vi "testInternalMemoryDispose.vi"(8 "error in (no error)":errorcluster, 11 "TestCase in":refnum<class "Memory Manager Unit Tests.lvclass">) -> (0 "error out":errorcluster, 3 "TestCase out":refnum<class "Memory Manager Unit Tests.lvclass">)   [LabVIEW 2016, in "Memory Manager Unit Tests.lvclass"]
uses:
  Memory Manager Unit Tests.lvclass
  Library/Classes/Pointer.Internal/Memory.Pointer.Internal.lvclass
  C:/Git/Personal/LabVIEW-Memory-Manager/Source/Library/Classes/Pointer/Memory.Pointer.lvclass
  Library/Classes/Pointer/Memory.Pointer.lvclass/Memory.Pointer.ctl
  Library/Classes/Pointer/Accessors/Get Address.vi
  <vilib>/addons/_JKI Toolkits/VI Tester/TestCase.llb/TestCase.lvclass
  C:/Program Files (x86)/National Instruments/LabVIEW 2016/vi.lib/addons/_JKI Toolkits/VI Tester/TestCase.llb/TestCase.lvclass
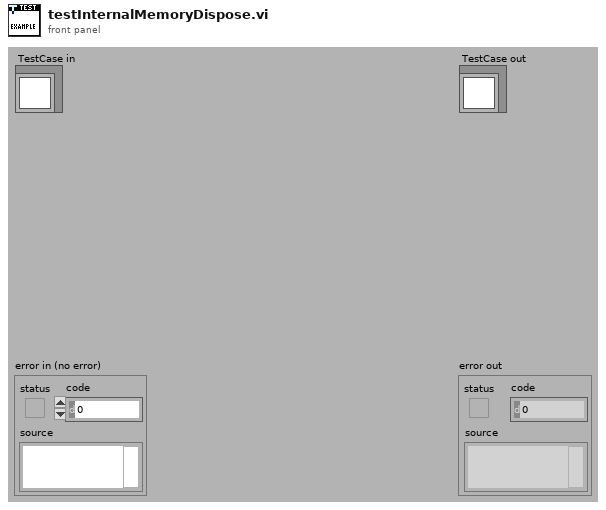
[diagram p1: front panel]
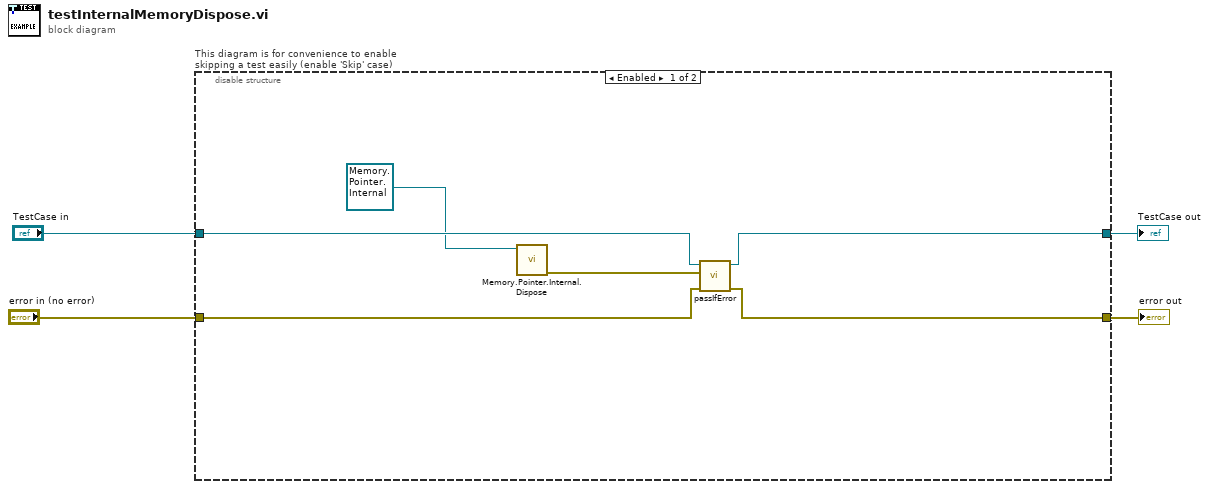
[diagram p0: block diagram]
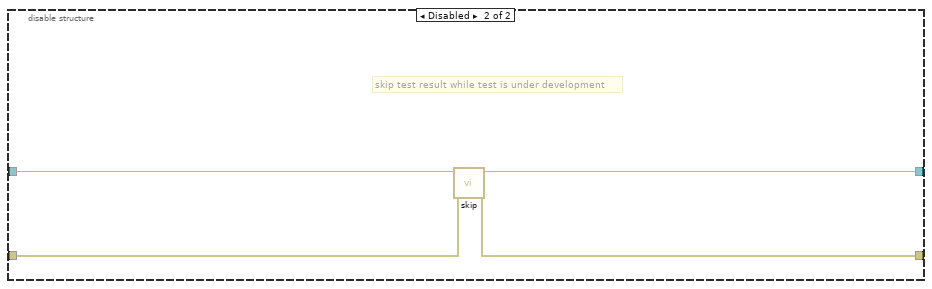
[diagram p2: hidden frame]
diagram:
  n1 = disable-structure "This diagram is for convenience to enable skipping a test easily (enable 'Skip' case)" shown="Enabled" {
    disable-tunnel: "TestCase in" -> [w10 w14]
    disable-tunnel: [w9 w12] -> w1
    disable-tunnel: [w8 w13] -> w3
    disable-tunnel: "error in (no error)" -> [w7 w11]
    frame Enabled {
      n2 = call "Memory.Pointer.Internal.Dispose.vi"("pointer"=refnum<class "Memory.Pointer.Internal.lvclass"> refnum) -> ("error out"=w6:errorcluster)  [unwired: 10 in]
      n3 = call-dynamic "passIfError.vi"("error in (no error)"=w7, "error"=w6, "TestCase in"=w10) -> ("error out"=w8:errorcluster, "TestCase out"=w9:refnum<class "Memory Manager Unit Tests.lvclass">)  [unwired: 7 in]
    }
    frame Disabled {
      # "skip test result while test is under development"
      n4 = call <vilib>:"skip.vi"("error in (no error)"=w11, "TestCase in"=w14) -> ("error out"=w13:errorcluster, "TestCase out"=w12:refnum<class "Memory Manager Unit Tests.lvclass">)  [unwired: 8 in]
    }
  }
  "error out" <- w3
  "TestCase out" <- w1
